vi "NI start task.vi"(8 "error in (no error)":errorcluster, 11 "NI in":refnum<class "NI.lvclass">) -> (0 "error out":errorcluster, 3 "NI out":refnum<class "NI.lvclass">)   [LabVIEW 2021, in "NI.lvlib" / "NI.lvclass"]
uses:
  NI.lvclass
  C:/Program Files (x86)/National Instruments/LabVIEW 2021/vi.lib/ActorFramework/Actor/Actor.lvclass
  NI.lvclass/NI.ctl
  Main_Control/Main_Control/notifications.ctl
  <vilib>/ActorFramework/Actor/Actor.lvclass/Actor.ctl
  Main_Control/Main_Control Messages/UI notifier Msg/UI notifier Msg.lvclass/UI notifier Msg.ctl
  <vilib>/ActorFramework/Message Enqueuer/Message Enqueuer.lvclass/Message Enqueuer.ctl
  <vilib>/ActorFramework/Message Enqueuer/Enqueue.vi
  Main_Control/Main_Control Messages/UI notifier Msg/UI notifier Msg.lvclass
  C:/Program Files (x86)/National Instruments/LabVIEW 2021/vi.lib/ActorFramework/Message/Message.lvclass
  <vilib>/ActorFramework/Message Priority Queue/Priority Enqueue.vi
  <vilib>/ActorFramework/Actor/Actor.lvclass
  Main_Control/Main_Control/Main_Control.lvclass
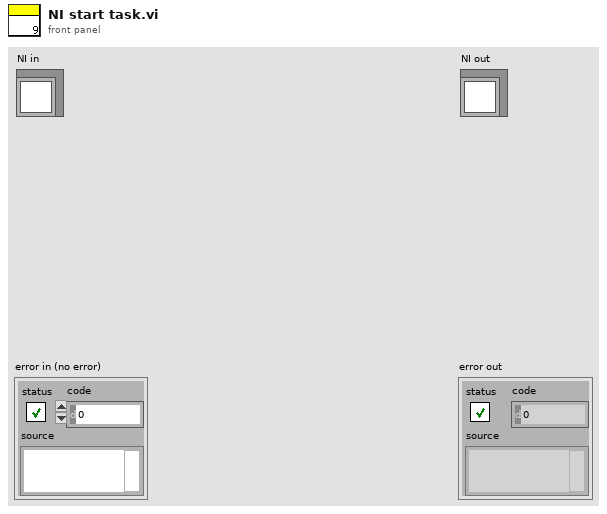
[diagram p1: front panel]
types:
  T1 = typedef "Main_Control.lvlib/Main_Control.lvclass/notifications.ctl" = enum16{"cam 1 frame skkipped", "cam finish", "cam started", "cam stopped", "cam updated", "ni started", "ni stopped", "ni updated"}
  T2 = cluster{"AO1 laser":refnum<k21>, "AO2 zy":refnum<k21>, "CO1 mainTrig":refnum<k21>, "CO2 fastClock":refnum<k21>, "AI phase":refnum<k21>}
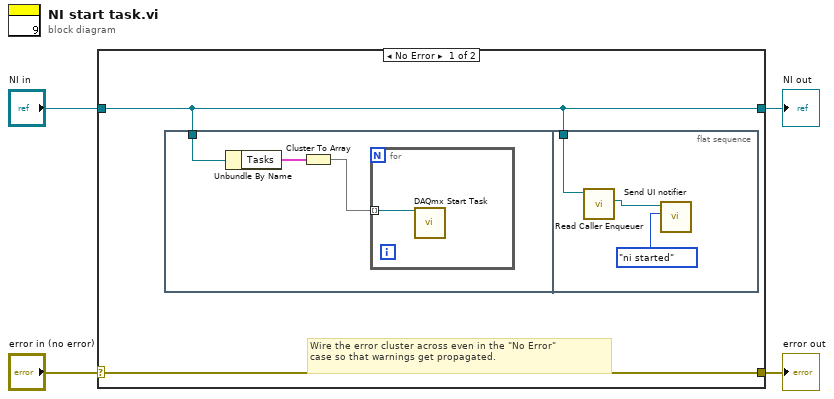
[diagram p0: block diagram]
diagram:
  n1 = case shown="No Error" "error in (no error)" {
    selector: "error in (no error)" -> [w6 w15]
    tunnel: [w6 w15] -> w3
    tunnel: [w5 w14] -> w1
    tunnel: "NI in" -> [w5 w14]
    frame No Error {
      # "Wire the error cluster across even in the \"No Error\"\ncase so that warnings get propagated."
      n2 = flat-sequence {
        tunnel: w5 -> [w9]
        tunnel: w5 -> [w13]
        frame #0 {
          n3 = Unbundle By Name(w9) -> ("Tasks"=w8:T2)
          n4 = Cluster To Array(cluster=w8) -> (array=w7:refnum<k21>[])
          n5 = for {
            tunnel: w7 -> [w10] mode=indexing
            n6 = call <vilib>:"DAQmx Start Task.vi"("task/channels in"=w10) -> ()  [unwired: 13 in, 2 out]
          }
        }
        frame #1 {
          n7 = call <vilib>:"Read Caller Enqueuer.vi"("Actor"=w13) -> ("Caller Enqueuer"=w11:refnum<class "Message Enqueuer.lvclass">)  [unwired: 10 in]
          n8 = call "Send UI notifier.vi"("Object&State"=notifications."ni started", "Message Enqueuer"=w11) -> ()  [unwired: 8 in, 2 out]
        }
      }
    }
    frame Error {
    }
  }
  "error out" <- w3
  "NI out" <- w1
